vi "ComponentInfos 2 Text.vi"(8 "Separator":string=" / ", 11 "Component Infos":T1) -> (3 "Component Text Array":T2[](array[typedef]))   [LabVIEW 2020, in "Linearisierung v2.lvlib" / "SpanEinstellungen.lvlib"]
uses:
  SpanEinstellungen.lvlib
  Visualisierungs Elemente/String - Ausgabefeld.ctl
  ComponentInfos.ctl
  Visualisierungs Elemente/String - Eingabefeld.ctl
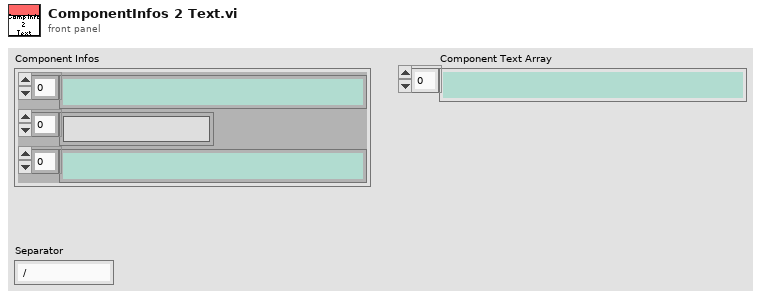
[diagram p1: front panel]
types:
  T1 = typedef "Linearisierung v2.lvlib/SpanEinstellungen.lvlib/ComponentInfos.ctl" = cluster{T2[], T3[], T2[]}
  T2 = typedef "String - Ausgabefeld.ctl" = string
  T3 = typedef "String - Eingabefeld.ctl" = string
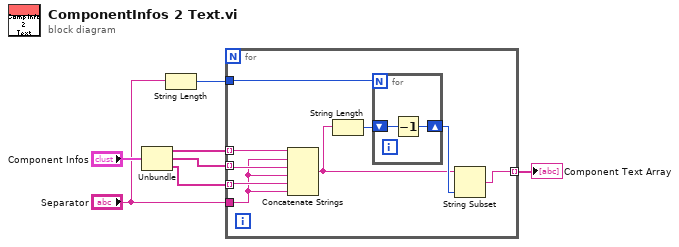
[diagram p0: block diagram]
diagram:
  n1 = Unbundle("Component Infos") -> (w6:T2[], w5:T3[], w4:T2[])
  n2 = String Length(string="Separator") -> (length=w1:i32)
  n3 = for {
    tunnel: w6 -> [w16] mode=indexing
    tunnel: w5 -> [w15] mode=indexing
    tunnel: w4 -> [w14] mode=indexing
    tunnel: "Separator" -> [w13]
    tunnel: [w9] -> w3 mode=indexing
    tunnel: w1 -> [w8]
    n4 = Concatenate Strings(w16, w13, w15, w13, w14, w13) -> (w10:string)
    n5 = String Length(string=w10) -> (length=w12:i32)
    n6 = for {
      N: w8 -> [_]
      shift-right: [w17] -> w11
      shift-left: w12 -> [w18]
      n7 = Decrement(x=w18) -> (x-1=w17:i32)
    }
    n8 = String Subset(string=w10, length (rest)=w11) -> (substring=w9:string)  [unwired: 1 in]
  }
  "Component Text Array" <- w3
